vi "Calculate TOP (Normal Mode).vi"(9 "Requested Frequency (Hz)":dbl, 10 "Clock Divisor":u32, 11 "Base Clock Frequency (Hz)":dbl) -> (2 "TOP":dbl, 3 "Remainder?":bool)   [LabVIEW 2021]
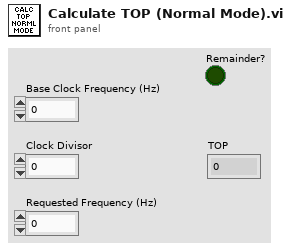
[diagram p1: front panel]
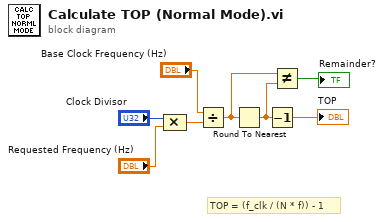
[diagram p0: block diagram]
diagram:
  # "TOP = (f_clk / (N * f)) - 1"
  n1 = Compound Arithmetic op=MULTIPLY("Clock Divisor", "Requested Frequency (Hz)") -> (w6:dbl)
  n2 = Divide(x="Base Clock Frequency (Hz)", y=w6) -> (x/y=w2:dbl)
  n3 = Round To Nearest(number=w2) -> (nearest integer value=w1:dbl)
  n4 = Decrement(x=w1) -> (x-1=→"TOP":dbl)
  n5 = Not Equal?(x=w2, y=w1) -> (x != y?=→"Remainder?":bool)
